vi "Soft_Stop_2017.vi"(0 "Hi Limit":dbl=35.0, 1 "Disable Motor":bool, 2 "Disable Softstops":bool, 3 "Motor Coerce":dbl=1.0, 5 "Lo Speed near Limit":dbl=0.02, 7 "Lo Limit":dbl=-10.0, 9 "Hi Speed near Limit":dbl=0.02, 11 "Lo Near Limit":dbl=1.0, 12 "Motor In":dbl=0.04, 13 "Sense":dbl, 14 "Hi Near Limit":dbl=1.0) -> (4 "At Hi":bool, 6 "At Lo":bool, 8 "Motor Out":dbl)   [LabVIEW 2016]
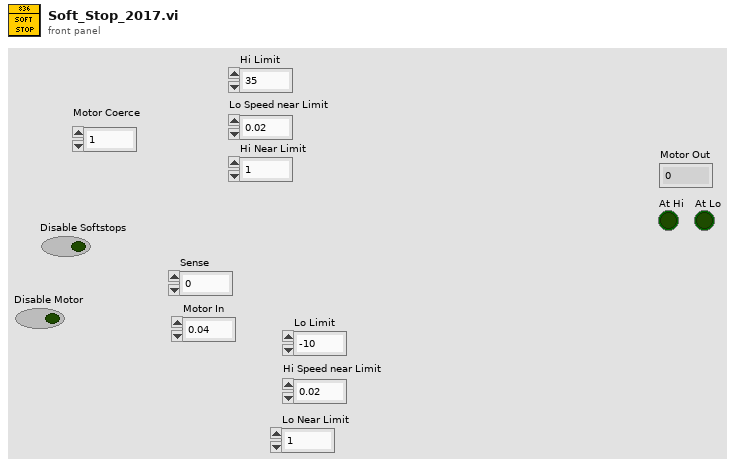
[diagram p1: front panel]
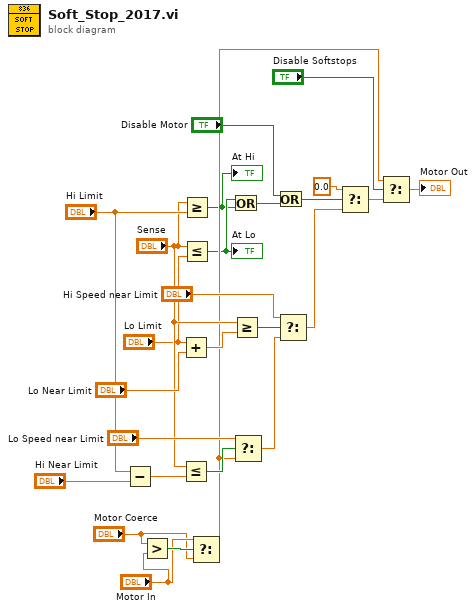
[diagram p0: block diagram]
diagram:
  n1 = Subtract(x="Hi Limit", y="Hi Near Limit") -> (x-y=w25:dbl)
  n2 = Greater?(x="Motor Coerce", y="Motor In") -> (0:w3:bool)
  n3 = Add(x="Lo Limit", y="Lo Near Limit") -> (x+y=w23:dbl)
  n4 = Less Or Equal?(x="Sense", y=w25) -> (x <= y?=w19:bool)
  n5 = Greater Or Equal?(x="Sense", y="Hi Limit") -> (x >= y?=w4:bool)
  "At Hi" <- w4
  n6 = Less Or Equal?(x="Sense", y="Lo Limit") -> (x <= y?=w5:bool)
  "At Lo" <- w5
  n7 = Select(t="Motor In", s=w3, f="Motor Coerce") -> (s? t:f=w7:dbl)
  n8 = Or(x=w5, y=w4) -> (x .or. y?=w12:bool)
  n9 = Greater Or Equal?(x="Sense", y=w23) -> (x >= y?=w18:bool)
  n10 = Select(t="Lo Speed near Limit", s=w19, f=w7) -> (s? t:f=w22:dbl)
  n11 = Or(x="Disable Motor", y=w12) -> (x .or. y?=w13:bool)
  n12 = Select(t="Hi Speed near Limit", s=w18, f=w22) -> (s? t:f=w17:dbl)
  n13 = Select(t=0.0, s=w13, f=w17) -> (s? t:f=w8:dbl)
  n14 = Select(t=w7, s="Disable Softstops", f=w8) -> (s? t:f=→"Motor Out":dbl)
